vi "Heartbeat Message to JSON.vi"(2 "error in":errorcluster, 3 "Heartbeat Message":T1) -> (0 "error out":errorcluster, 1 "JSON string":string)   [LabVIEW 2016]
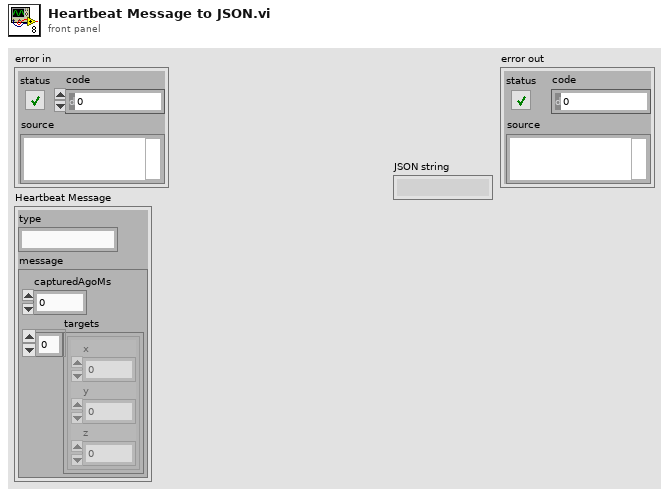
[diagram p1: front panel]
types:
  T1 = cluster{"type":string, "message":cluster{"capturedAgoMs":i32, "targets":cluster{"x":dbl, "y":dbl, "z":dbl}[]}}
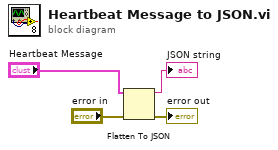
[diagram p0: block diagram]
diagram:
  n1 = Flatten To JSON(anything="Heartbeat Message", error in (no error)="error in") -> (JSON string=→"JSON string":string, 11:→"error out":errorcluster)  [unwired: 1 in]
